vi "TCP-IP Q_Bridge.Add Msg 4 Byte Length Header, I32.vi"(11 "Message":string) -> (3 "Message + Header":string)   [LabVIEW 2024, in "EQMF.lvlib" / "TCP-IP.lvlib"]
uses:
  TCP-IP.lvlib
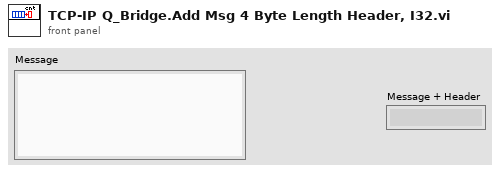
[diagram p1: front panel]
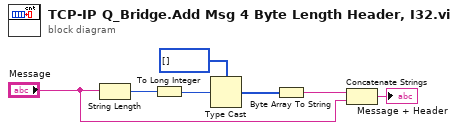
[diagram p0: block diagram]
diagram:
  n1 = String Length(string="Message") -> (length=w5:i32)
  n2 = To Long Integer(number=w5) -> (32bit integer=w7:i32)
  n3 = Type Cast(type=u8[] [], x=w7) -> (*(type *) &x=w4:u8[])
  n4 = Byte Array To String(unsigned byte array=w4) -> (string=w1:string)
  n5 = Concatenate Strings(w1, "Message") -> (→"Message + Header":string)
